vi "Global.vi"() -> ()   [LabVIEW 2012]
panel:
  in  "IsNotFind":bool
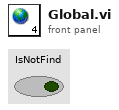
[diagram p1: front panel]
diagram:
